vi "niRFUtil CAL Calibration Data to List.vi"(9 "Calibration Data":T1 {"Calibration Table" min=0 max=127 format="%.2p"; "Time Stamp (sec)" format="%^.2e"; "Temperature (C)" format="%.1f"}) -> (1 "List":string[][](array[string]))   [LabVIEW 2015, in "niRFUtil.lvlib"]
uses:
  niRFUtil.lvlib
  Includes/niRFUtil INC Calibration Data.ctl
  Includes/niRFUtil INC Calibration Table.ctl
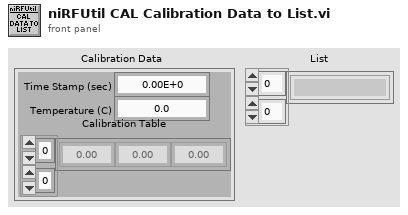
[diagram p1: front panel]
types:
  T1 = typedef "niRFUtil.lvlib/niRFUtil INC Calibration Data.ctl" = cluster{"Temperature (C)":dbl, "Time Stamp (sec)":dbl, "Calibration Table":T2}
  T2 = typedef "niRFUtil.lvlib/niRFUtil INC Calibration Table.ctl" = sgl[][]
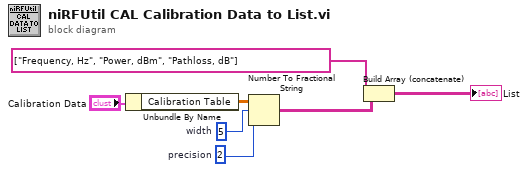
[diagram p0: block diagram]
diagram:
  w5 = 2  # precision
  w4 = 5  # width
  n1 = Unbundle By Name("Calibration Data") -> ("Calibration Table"=w2:T2)
  n2 = Number To Fractional String(number=w2, width (-)=w4, precision (6)=w5) -> (F-format string=w1:string[][])  [unwired: 1 out]
  n3 = Build Array (concatenate)(string[] ["Frequency, Hz", "Power, dBm", "Pathloss, dB"] ("array"), w1) -> (→"List":string[][])
